vi "FR Do Single Measurement.vi"(6 "Iteration index":i32, 7 "TWM handle in":i32, 8 "error in (no error)":errorcluster, 9 "FR measurement":T4={"Measurement frequencies (Hz)"=[1000.0, 10000.0, 1000.0], "Sampling frequency (Hz)"=500000.0, "Signal amplitude (V)"=4.5, "AC-DC settle time (s)"=20.0, "Record length (multiples of period)"=[1000.0, 10000.0, 1000.0], "Measurement template file"=path "", "Row of START keyword"=0, "Row of STOP keyword"=0, "Calculate RMS from samples"=FALSE, "AC-DC warm up time (s)"=300.0, "Measurement template line"=[], "DC meter readings No."=10, "Algorithm"="TWM-WFFT", "Simultaneous measurement"=FALSE, "Recalculate-skip already calculated"=FALSE} {"Record length (multiples of period)" format="%#_3p"; "Sampling frequency (Hz)" format="%#_3p"; "Measurement frequencies (Hz)" format="%#_3p"}, 10 "Common properties":T3={"Measurement status ref"=refnum, "TWM Status ref"=refnum, "Abort ref"=refnum, "Skip waiting ref"=refnum, "GNU Octave path"=path "C:/Program Files/GNU Octave/Octave-6.2.0/mingw64/bin", "TWM+QWTB path"=path "C:/Users/labina/Desktop/TWM-1.8.7.0-full/octprog", "lvlib path"=path "D:/martin/WAC/WACsw - github/control_software/Filter function meter/external libraries/GOLPI 0.7.3.1 source distribution LV 20.0 32 bit/lv_proc.dll", "TWM pipe"="\\\\.\\pipe\\TWM:server", "PJVS status ref"=refnum, "WAC path"=path ""}, 11 "DC meter":T1={"DC meter type"=enum."H/A/K 3458", "DC meter VISA"="", "NPLC"=10.0, "status ref"=refnum}) -> (0 "error out":errorcluster, 1 "TWM result as string":string[][](array[string]), 2 "DC readings":dbl[](array[numeric]), 3 "DC meter out":T1={"DC meter type"=enum."H/A/K 3458", "DC meter VISA"="", "NPLC"=10.0, "status ref"=refnum}, 5 "TWM handle out":i32)   [LabVIEW 2020]
doc: "Makes a single measurement in TWM and multimeter DC readings. Either in parallel, or in series. Setup TWM for single FR measurement, start TWM and read output, read out DC meter."
uses:
  Type definitions/FR measuement.ctl
  Utilities/Type definitions/Common properties.ctl
  General DC meter/Type definitions/DC meter.ctl
  General DC meter/Type definitions/DC meter type.ctl
  Utilities/Type definitions/Sampling properties.ctl
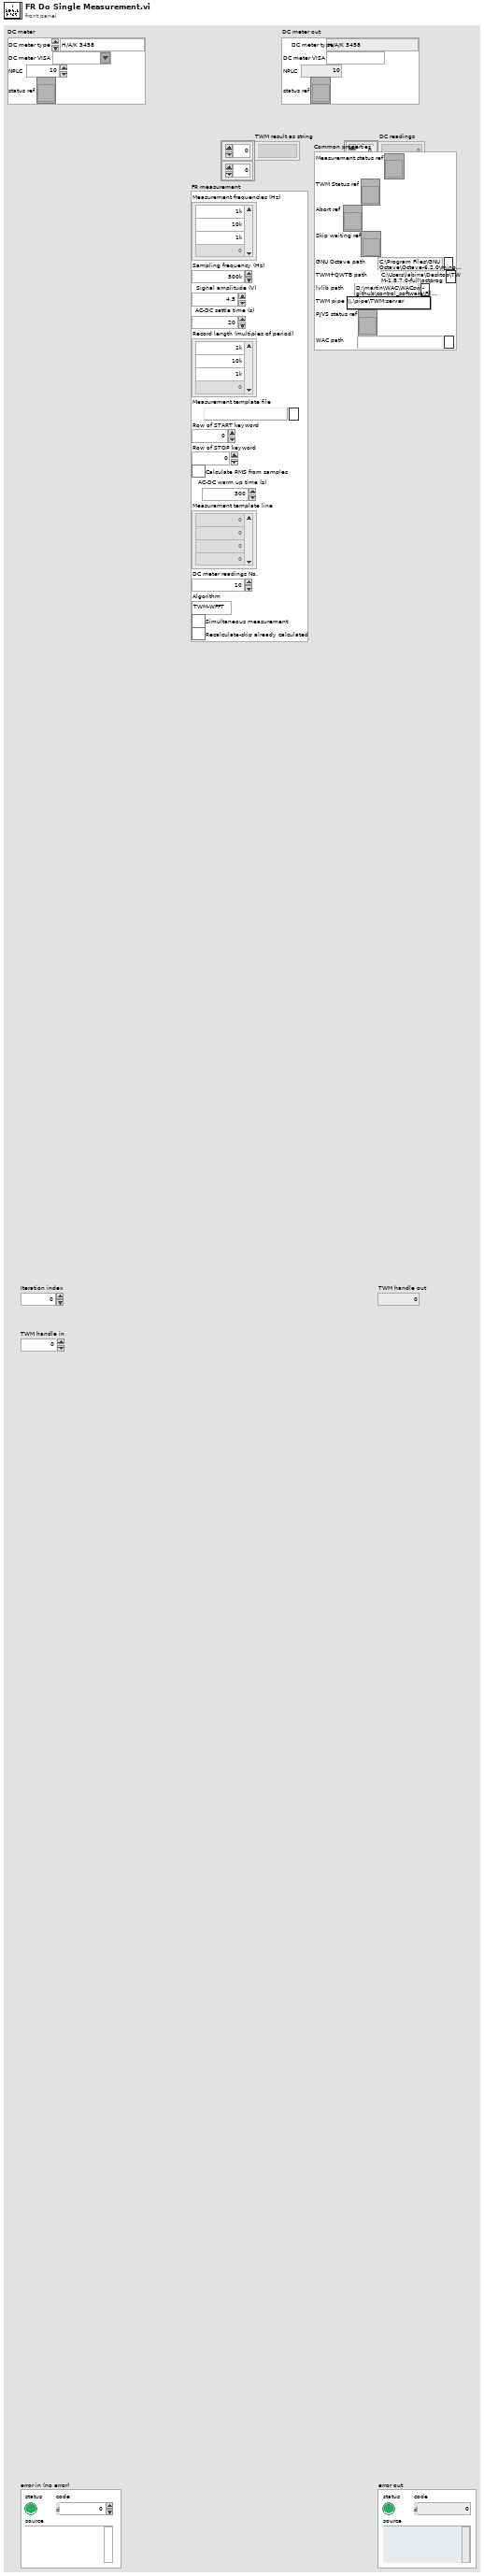
[diagram p1: front panel]
types:
  T1 = typedef "DC meter.ctl" = cluster{"DC meter type":T2, "DC meter VISA":refnum<visa-resource-name>, "NPLC":dbl, "status ref":refnum<vi>}
  T2 = typedef "DC meter type.ctl" = enum16{"H/A/K 3458", "Fluke 8508A", "dummy", "Keithley 2182"}
  T3 = typedef "Common properties.ctl" = cluster{"Measurement status ref":refnum<vi>, "TWM Status ref":refnum<vi>, "Abort ref":refnum<vi>, "Skip waiting ref":refnum<vi>, "GNU Octave path":path, "TWM+QWTB path":path, "lvlib path":path, "TWM pipe":string, "PJVS status ref":refnum<vi>, "WAC path":path}
  T4 = typedef "FR measuement.ctl" = cluster{"Measurement frequencies (Hz)":dbl[], "Sampling frequency (Hz)":dbl, "Signal amplitude (V)":dbl, "AC-DC settle time (s)":dbl, "Record length (multiples of period)":dbl[], "Measurement template file":path, "Row of START keyword":i32, "Row of STOP keyword":i32, "Calculate RMS from samples":bool, "AC-DC warm up time (s)":dbl, "Measurement template line":i32[], "DC meter readings No.":i32, "Algorithm":string, "Simultaneous measurement":bool, "Recalculate-skip already calculated":bool}
  T5 = typedef "Sampling properties.ctl" = cluster{"Sampling frequency (Hz)":dbl, "Record length (multiples of period)":dbl, "Signal amplitude (V)":dbl, "Measurement frequency (Hz)":dbl, "Calculate RMS from samples":bool, "Algorithm":string, "Measurement path":string}
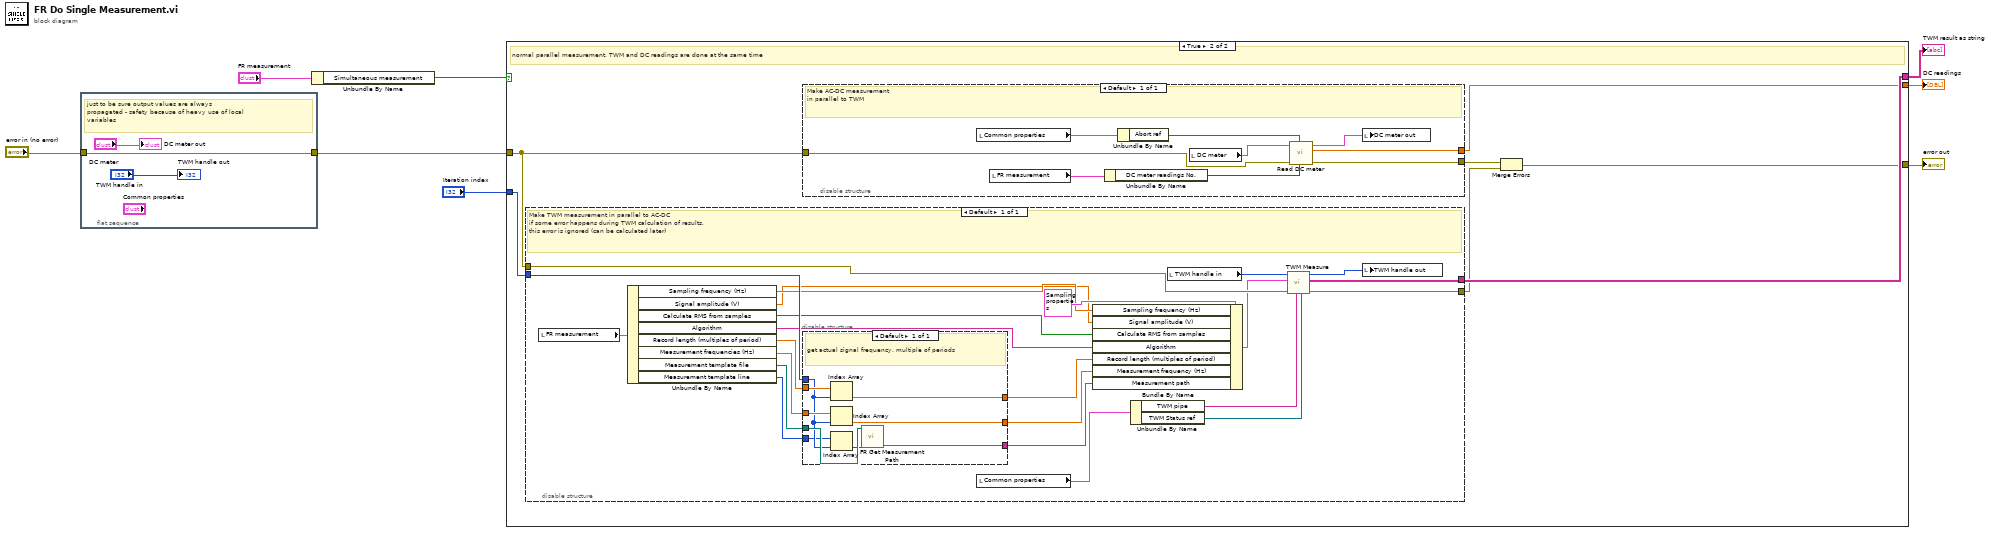
[diagram p0: block diagram]
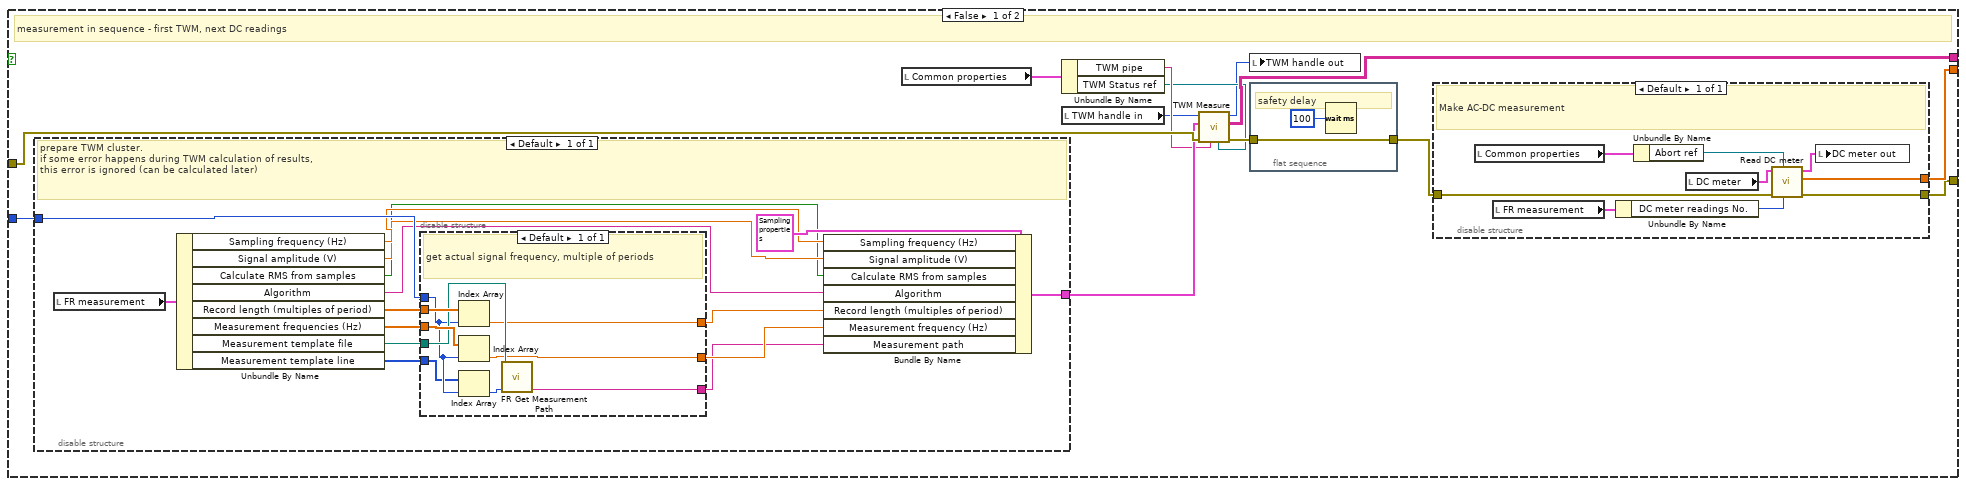
[diagram p2: hidden frame]
diagram:
  n1 = flat-sequence {
    tunnel: [w9] -> w2
    tunnel: "error in (no error)" -> [w9]
    frame #0 {
      # "just to be sure output values are always \npropagated - safety because of heavy use of local\nvariables"
      "TWM handle out" <- "TWM handle in"
      "DC meter out" <- "DC meter"
    }
  }
  n2 = Unbundle By Name("FR measurement") -> ("Simultaneous measurement"=w3:bool)
  n3 = case shown="True" w3 {
    tunnel: "Iteration index" -> [w24 w66]
    tunnel: [w17 w65] -> w7
    tunnel: [w23 w64] -> w6
    tunnel: w2 -> [w20 w63]
    tunnel: [w22 w60] -> w5
    frame False {
      # "measurement in sequence - first TWM, next DC readings"
      n4 = disable-structure shown="Default" {
        disable-tunnel: w24 -> [w49]
        disable-tunnel: [w45] -> w19
        frame Enabled {
          # "prepare TWM cluster.\nif some error happens during TWM calculation of results,\nthis error is ignored (can be calculated later)"
          n5 = local read "FR measurement"() -> (w36:T4)
          n6 = Unbundle By Name(w36) -> ("Sampling frequency (Hz)"=w44:dbl, "Signal amplitude (V)"=w43:dbl, "Calculate RMS from samples"=w42:bool, "Algorithm"=w41:string, "Record length (multiples of period)"=w40:dbl[], "Measurement frequencies (Hz)"=w39:dbl[], "Measurement template file"=w38:path, "Measurement template line"=w37:i32[])
          n7 = disable-structure shown="Default" {
            disable-tunnel: w39 -> [w59]
            disable-tunnel: w40 -> [w58]
            disable-tunnel: w49 -> [w55]
            disable-tunnel: [w57] -> w46
            disable-tunnel: w38 -> [w56]
            disable-tunnel: w37 -> [w54]
            disable-tunnel: [w52] -> w48
            disable-tunnel: [w51] -> w47
            frame Enabled {
              # "get actual signal frequency, multiple of periods"
              n8 = Index Array(array=w58, index=w55) -> (element=w51:dbl)
              n9 = Index Array(array=w59, index=w55) -> (element=w52:dbl)
              n10 = Index Array(array=w54, index=w55) -> (element=w53:i32)
              n11 = call "FR Get Measurement Path.vi"("Template line"=w53, "Measurement template file"=w56) -> ("Measurement path as string"=w57:string)  [unwired: 8 in, 1 out]
            }
          }
          n12 = Bundle By Name(cluster=T5 {"Sampling frequency (Hz)"=500000.0, "Record length (multiples of period)"=1000.0, "Signal amplitude (V)"=4.5, "Measurement frequency (Hz)"=1000.0, "Calculate RMS from samples"=FALSE, "Algorithm"="TWM-WFFT", "Measurement path"=""} ("TWM Measurement properties"), "Sampling frequency (Hz)"=w44, "Signal amplitude (V)"=w43, "Calculate RMS from samples"=w42, "Algorithm"=w41, "Record length (multiples of period)"=w47, "Measurement frequency (Hz)"=w48, "Measurement path"=w46) -> (w45:T5)
        }
      }
      n13 = local read "Common properties"() -> (w14:T3)
      n14 = Unbundle By Name(w14) -> ("TWM pipe"=w16:string, "TWM Status ref"=w15:refnum<vi>)
      n15 = local read "TWM handle in"() -> (w13:i32)
      n16 = call "TWM Measure.vi"("TWM Status ref"=w15, "TWM pipe"=w16, "error in (no error)"=w20, "TWM Measurement properties"=w19, "TWM handle"=w13) -> ("error out"=w18:errorcluster, "TWM result as string"=w17:string[][], "TWM handle out"=w12:i32)  [unwired: 3 in, 1 out]
      n17 = local write "TWM handle out"(w12) -> ()
      n18 = flat-sequence {
        tunnel: [w25] -> w21
        tunnel: w18 -> [w25]
        frame #0 {
          # "safety delay"
          n19 = Wait (ms)(milliseconds to wait=u32 100) -> ()  [unwired: 1 out]
        }
      }
      n20 = disable-structure shown="Default" {
        disable-tunnel: [w35] -> w23
        disable-tunnel: [w34] -> w22
        disable-tunnel: w21 -> [w33]
        frame Enabled {
          # "Make AC-DC measurement"
          n21 = local read "Common properties"() -> (w32:T3)
          n22 = local read "FR measurement"() -> (w30:T4)
          n23 = Unbundle By Name(w30) -> ("DC meter readings No."=w29:i32)
          n24 = Unbundle By Name(w32) -> ("Abort ref"=w31:refnum<vi>)
          n25 = local read "DC meter"() -> (w28:T1)
          n26 = call "Read DC meter.vi"("No of readings"=w29, "abort reference"=w31, "error in (no error)"=w33, "DC meter"=w28) -> ("error out"=w34:errorcluster, "DC readings"=w35:dbl[], "DC meter out"=w27:T1)  [unwired: 5 in]
          n27 = local write "DC meter out"(w27) -> ()
        }
      }
    }
    frame True {
      # "normal parallel measurement, TWM and DC readings are done at the same time"
      n28 = disable-structure shown="Default" {
        disable-tunnel: [w96] -> w61
        disable-tunnel: w63 -> [w98]
        disable-tunnel: w66 -> [w93]
        disable-tunnel: [w97] -> w65
        frame Enabled {
          # "Make TWM measurement in parallel to AC-DC\nif some error happens during TWM calculation of results,\nthis error is ignored (can be calculated later)"
          n29 = local read "FR measurement"() -> (w78:T4)
          n30 = Unbundle By Name(w78) -> ("Sampling frequency (Hz)"=w89:dbl, "Signal amplitude (V)"=w88:dbl, "Calculate RMS from samples"=w87:bool, "Algorithm"=w86:string, "Record length (multiples of period)"=w85:dbl[], "Measurement frequencies (Hz)"=w84:dbl[], "Measurement template file"=w83:path, "Measurement template line"=w82:i32[])
          n31 = disable-structure shown="Default" {
            disable-tunnel: w84 -> [w107]
            disable-tunnel: w85 -> [w106]
            disable-tunnel: w93 -> [w103]
            disable-tunnel: [w105] -> w90
            disable-tunnel: w83 -> [w104]
            disable-tunnel: w82 -> [w102]
            disable-tunnel: [w100] -> w92
            disable-tunnel: [w99] -> w91
            frame Enabled {
              # "get actual signal frequency, multiple of periods"
              n32 = Index Array(array=w106, index=w103) -> (element=w99:dbl)
              n33 = Index Array(array=w107, index=w103) -> (element=w100:dbl)
              n34 = Index Array(array=w102, index=w103) -> (element=w101:i32)
              n35 = call "FR Get Measurement Path.vi"("Template line"=w101, "Measurement template file"=w104) -> ("Measurement path as string"=w105:string)  [unwired: 8 in, 1 out]
            }
          }
          n36 = local read "Common properties"() -> (w81:T3)
          n37 = Bundle By Name(cluster=T5 {"Sampling frequency (Hz)"=500000.0, "Record length (multiples of period)"=1000.0, "Signal amplitude (V)"=4.5, "Measurement frequency (Hz)"=1000.0, "Calculate RMS from samples"=FALSE, "Algorithm"="TWM-WFFT", "Measurement path"=""} ("TWM Measurement properties"), "Sampling frequency (Hz)"=w89, "Signal amplitude (V)"=w88, "Calculate RMS from samples"=w87, "Algorithm"=w86, "Record length (multiples of period)"=w91, "Measurement frequency (Hz)"=w92, "Measurement path"=w90) -> (w94:T5)
          n38 = Unbundle By Name(w81) -> ("TWM pipe"=w80:string, "TWM Status ref"=w79:refnum<vi>)
          n39 = local read "TWM handle in"() -> (w76:i32)
          n40 = call "TWM Measure.vi"("TWM Status ref"=w79, "TWM pipe"=w80, "error in (no error)"=w98, "TWM Measurement properties"=w94, "TWM handle"=w76) -> ("error out"=w96:errorcluster, "TWM result as string"=w97:string[][], "TWM handle out"=w77:i32)  [unwired: 3 in, 1 out]
          n41 = local write "TWM handle out"(w77) -> ()
        }
      }
      n42 = disable-structure shown="Default" {
        disable-tunnel: [w75] -> w64
        disable-tunnel: [w74] -> w62
        disable-tunnel: w63 -> [w73]
        frame Enabled {
          # "Make AC-DC measurement\nin parallel to TWM"
          n43 = local read "Common properties"() -> (w72:T3)
          n44 = local read "FR measurement"() -> (w71:T4)
          n45 = Unbundle By Name(w71) -> ("DC meter readings No."=w69:i32)
          n46 = Unbundle By Name(w72) -> ("Abort ref"=w70:refnum<vi>)
          n47 = local read "DC meter"() -> (w68:T1)
          n48 = call "Read DC meter.vi"("No of readings"=w69, "abort reference"=w70, "error in (no error)"=w73, "DC meter"=w68) -> ("error out"=w74:errorcluster, "DC readings"=w75:dbl[], "DC meter out"=w67:T1)  [unwired: 5 in]
          n49 = local write "DC meter out"(w67) -> ()
        }
      }
      n50 = Merge Errors(w62, w61) -> (w60:errorcluster)
    }
  }
  "TWM result as string" <- w7
  "error out" <- w5
  "DC readings" <- w6
